vi "Convert Between String and Array.vi"(7 "Separator (|)":string="|", 10 "String Array":string[](array[string]), 11 "String":string) -> (2 "String":string, 3 "String Array":string[](array[string]))   [LabVIEW 2016, in "DataGrid.lvlib" / "DataGridView.lvclass"]
doc: "Converts between an array of strings to a string array separated by some delimiter. The pipe character is default.\n\nAlso converts from string to array.\n\nMike King\nAdvanced Functions Inc.\nJune 20, 2002"
uses:
  <userlib>/LabVIEWdotNetDataGrid/source/DataGridView/DataGridView.lvclass
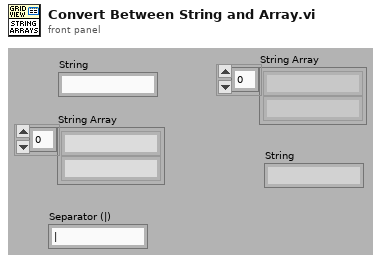
[diagram p1: front panel]
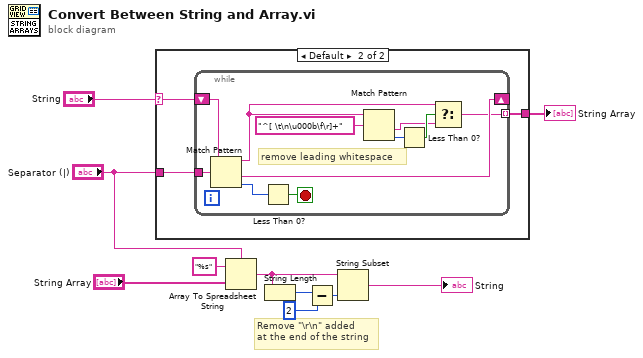
[diagram p0: block diagram]
diagram:
  # "Remove \"\\r\\n\" added\nat the end of the string"
  n1 = case shown="Default" "String" {
    selector: "String" -> [_ w11]
    tunnel: [_ w13] -> w10
    tunnel: "Separator (|)" -> [_ w12]
    frame "" {
    }
    frame Default {
      n2 = while {
        tunnel: [w14] -> w13 mode=indexing
        shift-left: w11 -> [w24]
        shift-right: [w23] -> _
        tunnel: w12 -> [w20]
        stop <- w22 stop-if-true
        # "remove leading whitespace"
        n3 = Match Pattern(string=w24, regular expression=w20) -> (before substring=w17:string, after substring=w23:string, offset past match=w21:i32)  [unwired: 1 in, 1 out]
        n4 = Less Than 0?(x=w21) -> (x < 0?=w22:bool)
        n5 = Match Pattern(string=w17, regular expression="^[ \t\n\u000b\f\r]+") -> (after substring=w16:string, offset past match=w15:i32)  [unwired: 1 in, 2 out]
        n6 = Less Than 0?(x=w15) -> (x < 0?=w19:bool)
        n7 = Select(t=w17, s=w19, f=w16) -> (s? t:f=w14:string)
      }
    }
  }
  "String Array" <- w10
  n8 = Array To Spreadsheet String(delimiter (Tab)="Separator (|)", array="String Array", 3:"%s" ("format string")) -> (spreadsheet string=w5:string)
  n9 = String Length(string=w5) -> (length=w4:i32)
  n10 = Subtract(x=w4, y=2) -> (x-y=w1:i32)
  n11 = String Subset(string=w5, length (rest)=w1) -> (substring=→"String":string)  [unwired: 1 in]
